vi "P22_Traffic.vi"() -> ()   [LabVIEW 2022 SP3]
panel:
  out "V1":bool
  out "A1":bool
  out "R1":bool
  out "R2":bool
  out "A2":bool
  out "V2":bool
  in  "stop":bool
  # "P22_Traffic"
  # "Equipo C\nJairo Issac García López\nRodolfo Durón Hernandez\nRoberto Carlos Herrera Pérez\nSebastián Rodríguez Posada"
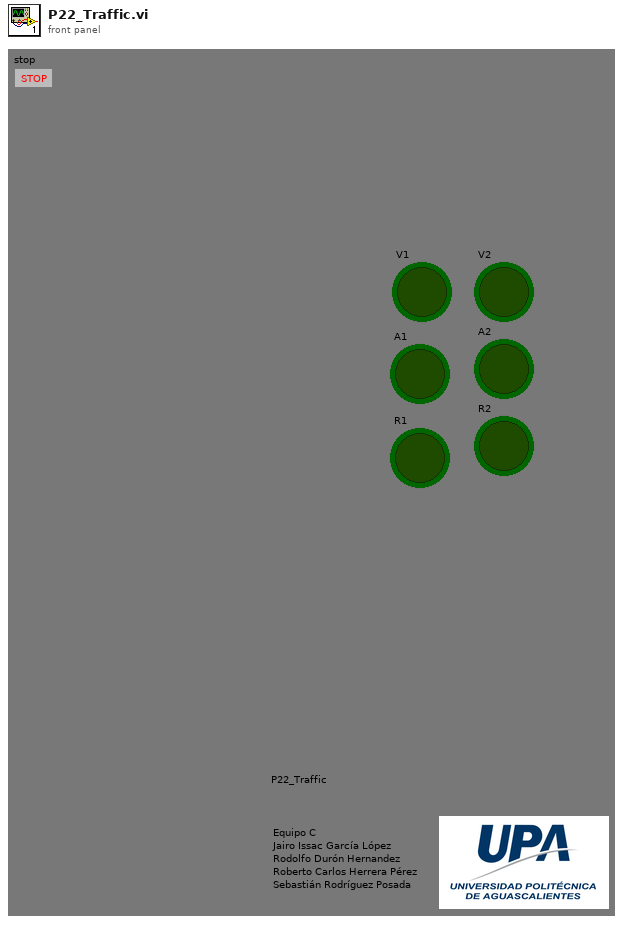
[diagram p1: front panel]
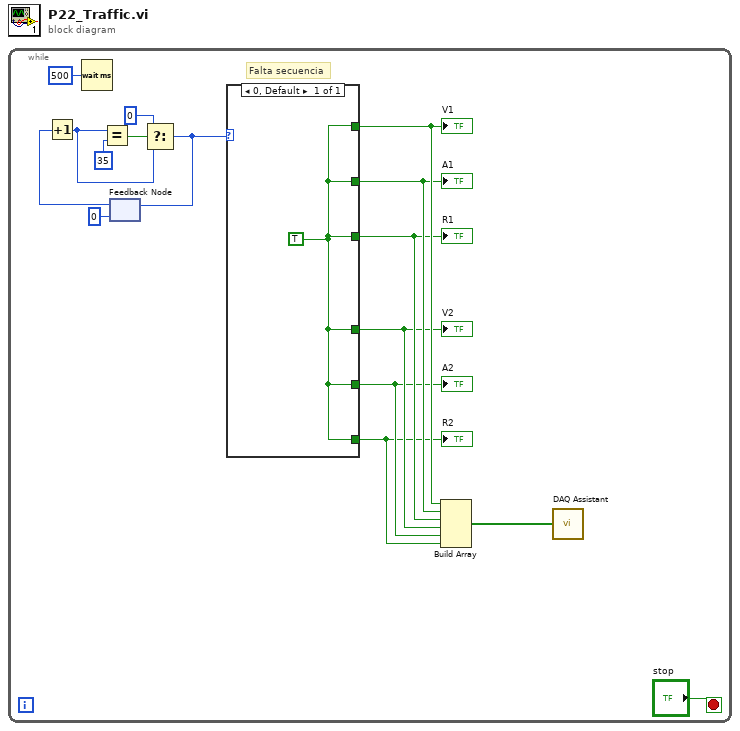
[diagram p0: block diagram]
diagram:
  n1 = while {
    stop <- "stop" stop-if-true
    # "Falta secuencia"
    n2 = Wait (ms)(milliseconds to wait=u32 500) -> ()  [unwired: 1 out]
    n3 = feedback #1(u8 0) -> (w13:u8)
    n4 = Increment(x=w13) -> (x+1=w10:u8)
    n5 = Equal?(x=w10, y=u8 35) -> (x = y?=w15:bool)
    n6 = Select(t=u8 0, s=w15, f=w10) -> (s? t:f=w9:u8)
    n7 = feedback-in #1(w9) -> ()
    n8 = case shown="0, Default" w9 {
      tunnel: [w17] -> w8
      tunnel: [w17] -> w7
      tunnel: [w17] -> w6
      tunnel: [w17] -> w5
      tunnel: [w17] -> w4
      tunnel: [w17] -> w3
      frame 0, Default {
        w17 = TRUE
      }
    }
    "V1" <- w8
    "A1" <- w7
    "R1" <- w6
    "R2" <- w3
    "A2" <- w4
    "V2" <- w5
    n9 = Build Array(w8, w7, w6, w5, w4, w3) -> (w2:bool[])
    n10 = call "DAQ Assistant"("data"=w2) -> ()  [unwired: 17 in, 2 out]
  }
